vi "LWXPS_PositionerAnalogTrackingPositionParametersSet.vi"(0 "Positioner Name":string, 1 "Analog input name":string, 2 "Offset":dbl, 3 "Scale":dbl, 4 "Velocity":dbl, 5 "Acceleration":dbl, 6 "XPS Reference IN":refnum<k24>, 7 "LabVIEW error IN":errorcluster) -> (14 "XPS Reference OUT":refnum<k24>, 15 "Returned error code":i32, 18 "XPS Error String":string, 19 "LabVIEW error OUT":errorcluster)   [LabVIEW 2015]
uses:
  D:/labview program/whole brain TP_220607/sub vi/XPS-UNIFIED/LabVIEW VIs/LabVIEW Source Code/Dll/Newport.XPS.CommandInterface.dll
  Dll/Newport.XPS.CommandInterface.dll
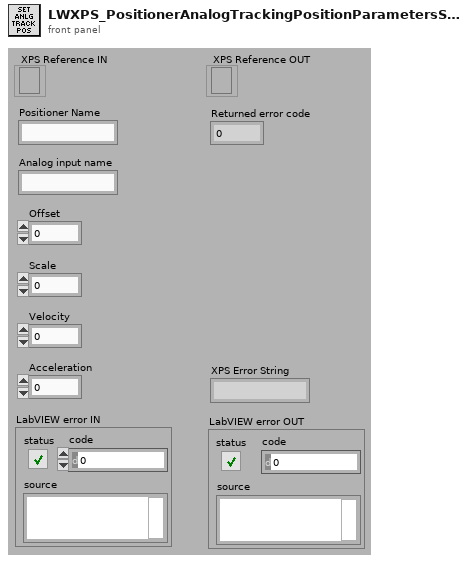
[diagram p1: front panel]
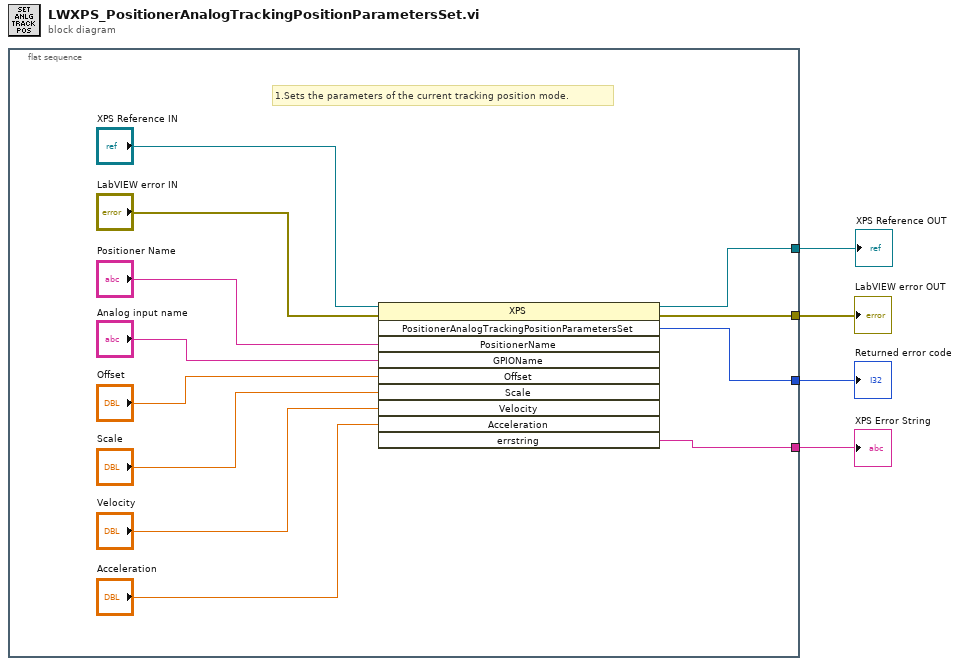
[diagram p0: block diagram]
diagram:
  n1 = flat-sequence {
    tunnel: [w12] -> w4
    tunnel: [w15] -> w3
    tunnel: [w14] -> w2
    tunnel: [w11] -> w1
    frame #0 {
      # "1.Sets the parameters of the current tracking position mode."
      n2 = invoke class="XPS" method="PositionerAnalogTrackingPositionParametersSet"(reference="XPS Reference IN", error in="LabVIEW error IN", "PositionerName"="Positioner Name", "GPIOName"="Analog input name", "Offset"="Offset", "Scale"="Scale", "Velocity"="Velocity", "Acceleration"="Acceleration") -> (reference out=w12:refnum<k24>, error out=w15:errorcluster, "PositionerAnalogTrackingPositionParametersSet"=w14:i32, "errstring"=w11:string)  [unwired: 2 in, 6 out]
    }
  }
  "XPS Error String" <- w1
  "XPS Reference OUT" <- w4
  "LabVIEW error OUT" <- w3
  "Returned error code" <- w2
